vi "Actor Core.vi"(8 "error in":errorcluster, 11 "DATABASE_MANEJO in":refnum<class "DATABASE_MANEJO.lvclass">) -> (0 "error out":errorcluster, 3 "Actor out":refnum<class "Actor.lvclass">)   [LabVIEW 2019, in "DATABASE_MANEJO.lvlib" / "DATABASE_MANEJO.lvclass"]
doc: "(<B>Filename</B>: Actor Framework.lvlib:Actor.lvclass:Actor Core.vi)\n\nReceives messages to the actor, reacts to them, and initiates any error handling that may shut the actor down.\n\nDescendant classes may override this VI to append parallel tasks for the actor to complete while it handles messages. Overrides use the Call Parent Method node."
uses:
  DATABASE_MANEJO.lvclass
  <vilib>/ActorFramework/Actor/Actor.lvclass
  DATABASE_MANEJO.lvclass/DATABASE_MANEJO.ctl
  <vilib>/drjdpowell/SQLite Library/SQL Connection/Open (path).vi
  <vilib>/drjdpowell/SQLite Library/SQL Connection/Open (string).vi
  <vilib>/AdvancedString/Path To Command Line String.vi
  <vilib>/drjdpowell/SQLite Library/SQL Connection/Execute SQL.vi
  <vilib>/drjdpowell/SQLite Library/SQL Connection/Connection.lvclass
  <vilib>/drjdpowell/SQLite Library/SQLite.lvlib
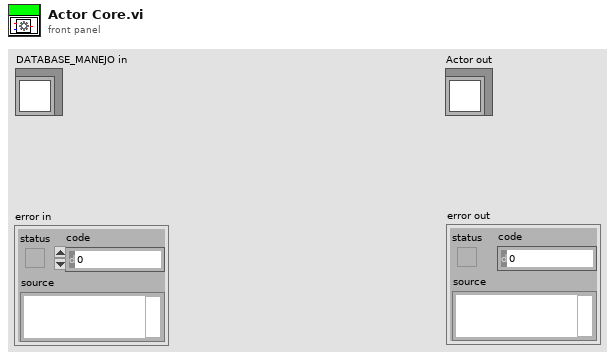
[diagram p1: front panel]
types:
  T1 = cluster{"Exit":refnum<user-event>, "BASE DE DATOS":refnum<user-event>}
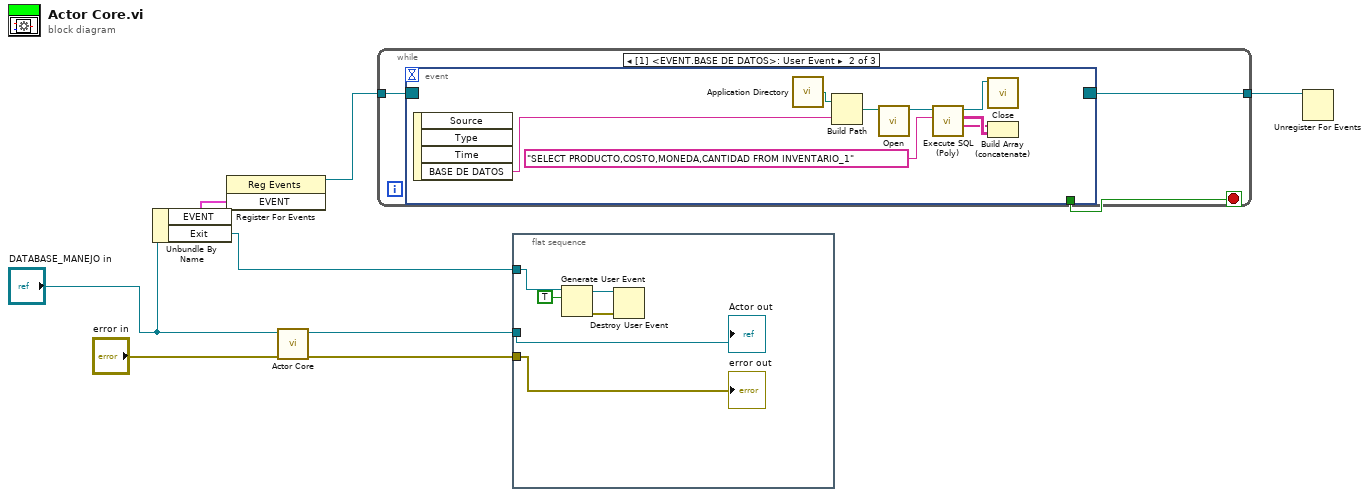
[diagram p0: block diagram]
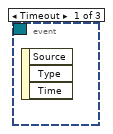
[diagram p2: hidden frame]
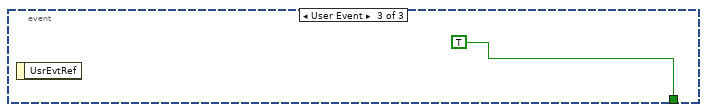
[diagram p3: hidden frame]
diagram:
  n1 = Unbundle By Name("DATABASE_MANEJO in") -> ("EVENT"=w6:T1, "Exit"=w2:refnum<user-event>)
  n2 = register-events(w6) -> (reference out=w5:refnum<event-registration>)  [unwired: 2 in, 1 out]
  n3 = call-parent "Actor Core.vi"("error in"="error in", "Actor in"="DATABASE_MANEJO in") -> ("error out"=w3:errorcluster, "Actor out"=w4:refnum<class "Actor.lvclass">)  [unwired: 8 in]
  n4 = while {
    tunnel: w5 -> [w11]
    tunnel: [w9] -> w1
    stop <- w10 stop-if-true
    n5 = event shown="[1] <EVENT.BASE DE DATOS>: User Event" {
      selector: w11 -> [_ _ _]
      dyn-events: [_ _ _] -> w9
      timeout: _ -> [_ _ _]
      tunnel: [_ _ TRUE] -> w10
      event Timeout {
        n6 = event-data() -> ()  [unwired: 1 in, 3 out]
      }
      event User Event {
        n7 = event-data() -> ("BASE DE DATOS"=w12:string)  [unwired: 1 in, 3 out]
        n8 = call <vilib>:"Application Directory.vi"() -> ("Application Directory"=w19:path)
        n9 = Build Path(base path=w19, name or relative path=w12) -> (appended path=w18:path)
        n10 = call-poly <vilib>:"Open.vi"("db file"=w18) -> ("SQLite Connection"=w17:refnum<class "Connection.lvclass">)  [unwired: 9 in, 1 out]
        n11 = call-poly <vilib>:"Execute SQL (Poly).vi"("SQL"="SELECT PRODUCTO,COSTO,MONEDA,CANTIDAD FROM INVENTARIO_1", "SQLite Connection in"=w17) -> ("Column Names"=w13:string[], "Result Set"=w14:string[][], "SQLite Connection"=w16:refnum<class "Connection.lvclass">)  [unwired: 6 in, 1 out]
        n12 = call-dynamic "Close.vi"("SQLite Connection in"=w16) -> ()  [unwired: 10 in, 1 out]
        n13 = Build Array (concatenate)(w13, w14) -> ()  [unwired: 1 out]
      }
      event User Event {
        n14 = event-data() -> ()  [unwired: 1 in, 1 out]
      }
    }
  }
  n15 = flat-sequence {
    tunnel: w4 -> [w26]
    tunnel: w3 -> [w25]
    tunnel: w2 -> [w24]
    frame #0 {
      n16 = Generate User Event(user event=w24, event data cluster=TRUE ("event data")) -> (user event out=w21:refnum<user-event>, error out=w22:errorcluster)  [unwired: 2 in]
      n17 = Destroy User Event(user event=w21, error in=w22) -> ()  [unwired: 1 out]
      "error out" <- w25
      "Actor out" <- w26
    }
  }
  n18 = Unregister For Events(event registration refnum=w1) -> ()  [unwired: 1 in, 1 out]
